vi "Rising Edge.vi"(11 "Input":bool) -> (3 "Rise?":bool)   [LabVIEW 2019]
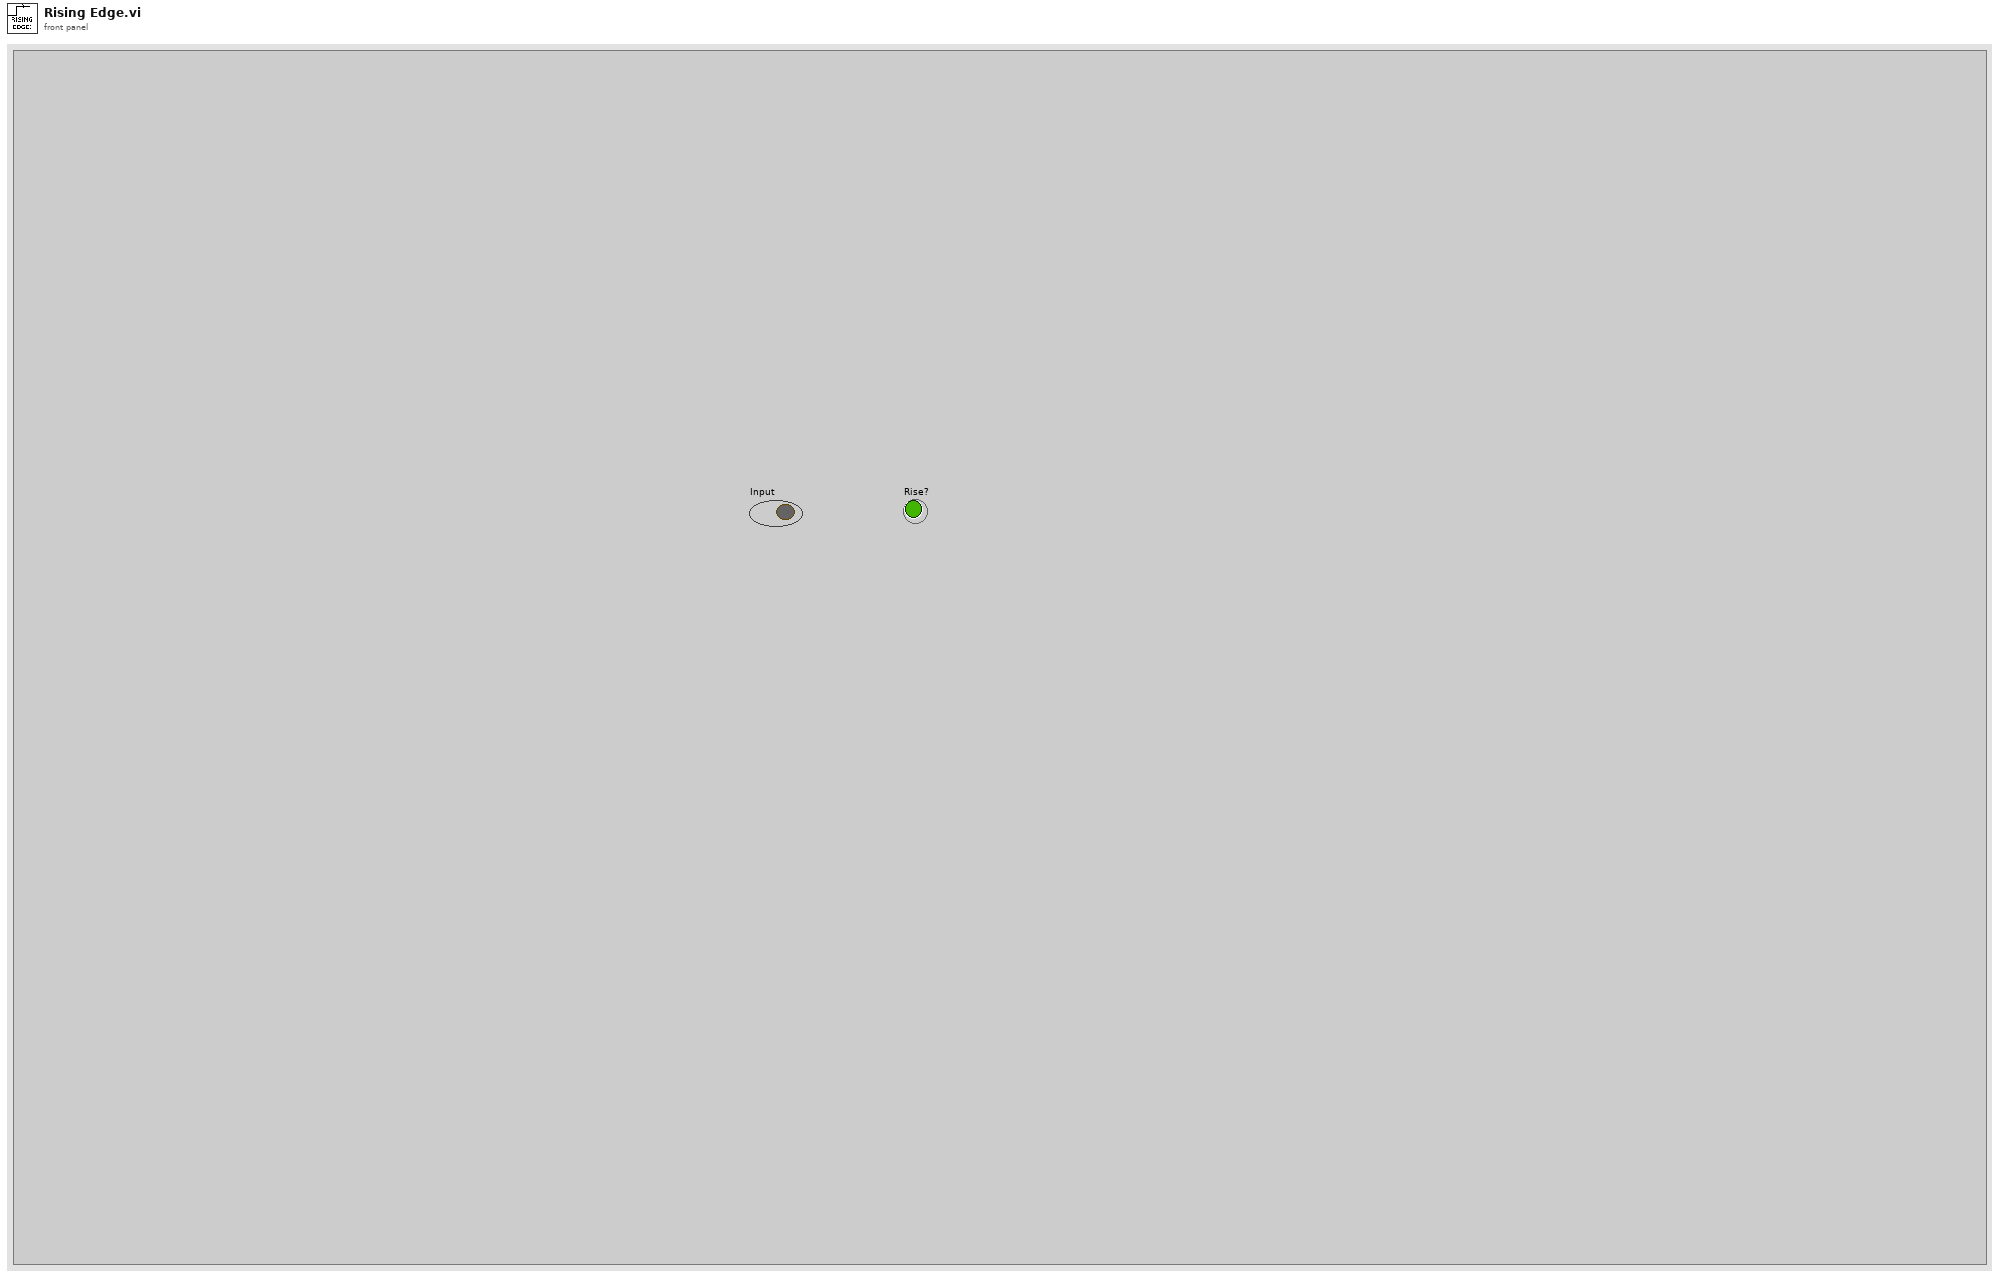
[diagram p1: front panel]
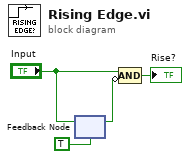
[diagram p0: block diagram]
diagram:
  n1 = feedback #1(TRUE) -> (w4:bool)
  n2 = feedback-in #1("Input") -> ()
  n3 = Compound Arithmetic op=AND("Input", invert w4) -> (→"Rise?":bool)
